vi "SN_Dialog.vi"() -> (2 "Cancelled":bool, 3 "UserName":string)   [LabVIEW 2022 SP3, in "Barcode_Reader_Dialog.lvlib" / "Barcode_Reader_Dialog.lvclass"]
uses:
  Barcode_Reader_Dialog.lvclass
panel:
  in  "SN":string caption="String"
  in  "OK":bool caption="Blank"
  in  "Cancel":bool caption="Blank"
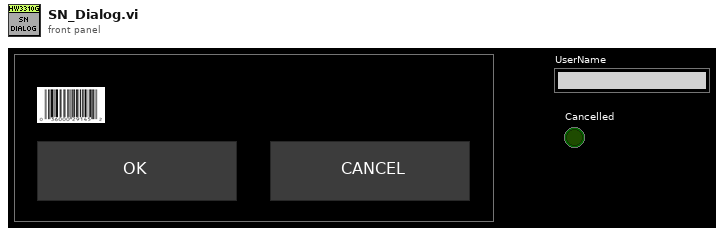
[diagram p1: front panel]
types:
  T1 = enum8{"Enabled", "Disabled", "Disabled and Grayed Out"}
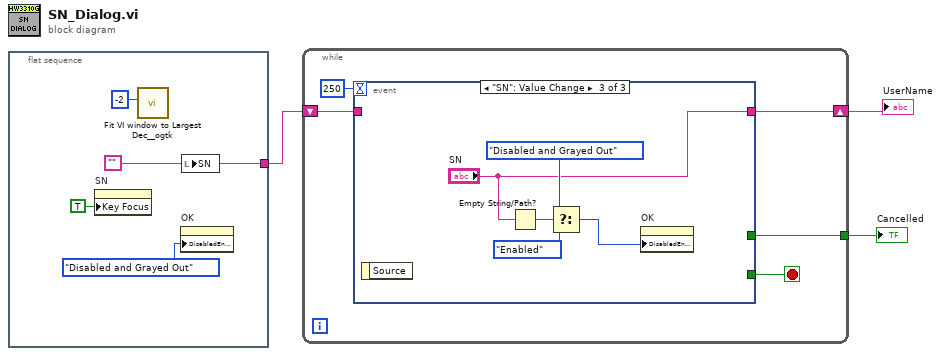
[diagram p0: block diagram]
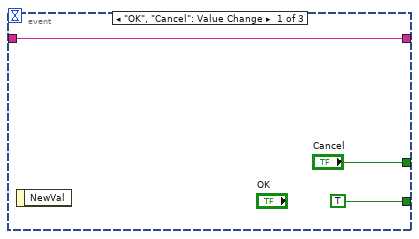
[diagram p2: hidden frame]
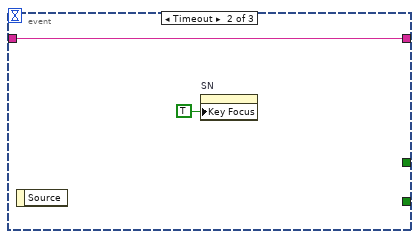
[diagram p3: hidden frame]
diagram:
  n1 = flat-sequence {
    tunnel: [w7] -> w2
    frame #0 {
      w7 = ""
      n2 = property on="SN" class="Str"("Key Focus"=TRUE) -> ()  [unwired: 2 in, 2 out]
      n3 = call <userlib>:"Fit VI window to Largest Dec__ogtk.vi"("border spacing (2 px)"=-2) -> ()  [unwired: 5 in, 2 out]
      n4 = property on="OK" class="Bool"("DisabledEnum"=T1."Disabled and Grayed Out" ("Disabled")) -> ()  [unwired: 2 in, 2 out]
      n5 = local write "SN"(w7) -> ()
    }
  }
  n6 = while {
    tunnel: [w11] -> w3
    shift-right: [w10] -> w1
    shift-left: w2 -> [w9]
    stop <- w12 stop-if-true
    n7 = event shown="[2] \"SN\": Value Change" {
      selector: _ -> [_ _ _]
      dyn-events: _ -> [_ _ _]
      timeout: 250 -> [_ _ _]
      tunnel: [TRUE ("OK") _ _] -> w12
      tunnel: ["Cancel" _ _] -> w11
      tunnel: [w13 w16 "SN"] -> w10
      tunnel: w9 -> [w13 w16 _]
      event "OK", "Cancel": Value Change {
        n8 = event-data() -> ()  [unwired: 1 in, 1 out]
      }
      event Timeout {
        n9 = event-data() -> ()  [unwired: 1 in, 1 out]
        n10 = property on="SN" class="Str"("Key Focus"=TRUE) -> ()  [unwired: 2 in, 2 out]
      }
      event "SN": Value Change {
        n11 = event-data() -> ()  [unwired: 1 in, 1 out]
        n12 = Empty String/Path?(string/path="SN") -> (empty?=w22:bool)
        n13 = Select(t=T1."Disabled and Grayed Out" ("Disabled"), s=w22, f=T1."Enabled" ("Disabled")) -> (s? t:f=w19:T1)
        n14 = property on="OK" class="Bool"("DisabledEnum"=w19) -> ()  [unwired: 2 in, 2 out]
      }
    }
  }
  "Cancelled" <- w3
  "UserName" <- w1
